vi "Labview_forward_pass.vi"() -> ()   [LabVIEW 2020]
uses:
  <vilib>/Analysis/NI_AALBase.lvlib
  <vilib>/Analysis/Matrix/NI_Matrix.lvlib
  <vilib>/Analysis/baseanly.llb/Real Dot Product.vi
  <vilib>/Analysis/Matrix/Numeric/Conversions/Array To Matrix - RA2.vi
  <vilib>/Analysis/baseanly.llb/Vector x A.vi
panel:
  out "i":i32
  out "xx":dbl[](array[numeric])
  out "element out":dbl
  out "XY Graph 2":cluster{i32[], dbl[]}(graph)
  out "y":dbl
  out "Array":i32[](array[numeric])
  out "XY Graph":T1(graph)
  out "X":dbl[](graph)
  out "All input data":waveform(dbl)(graph)
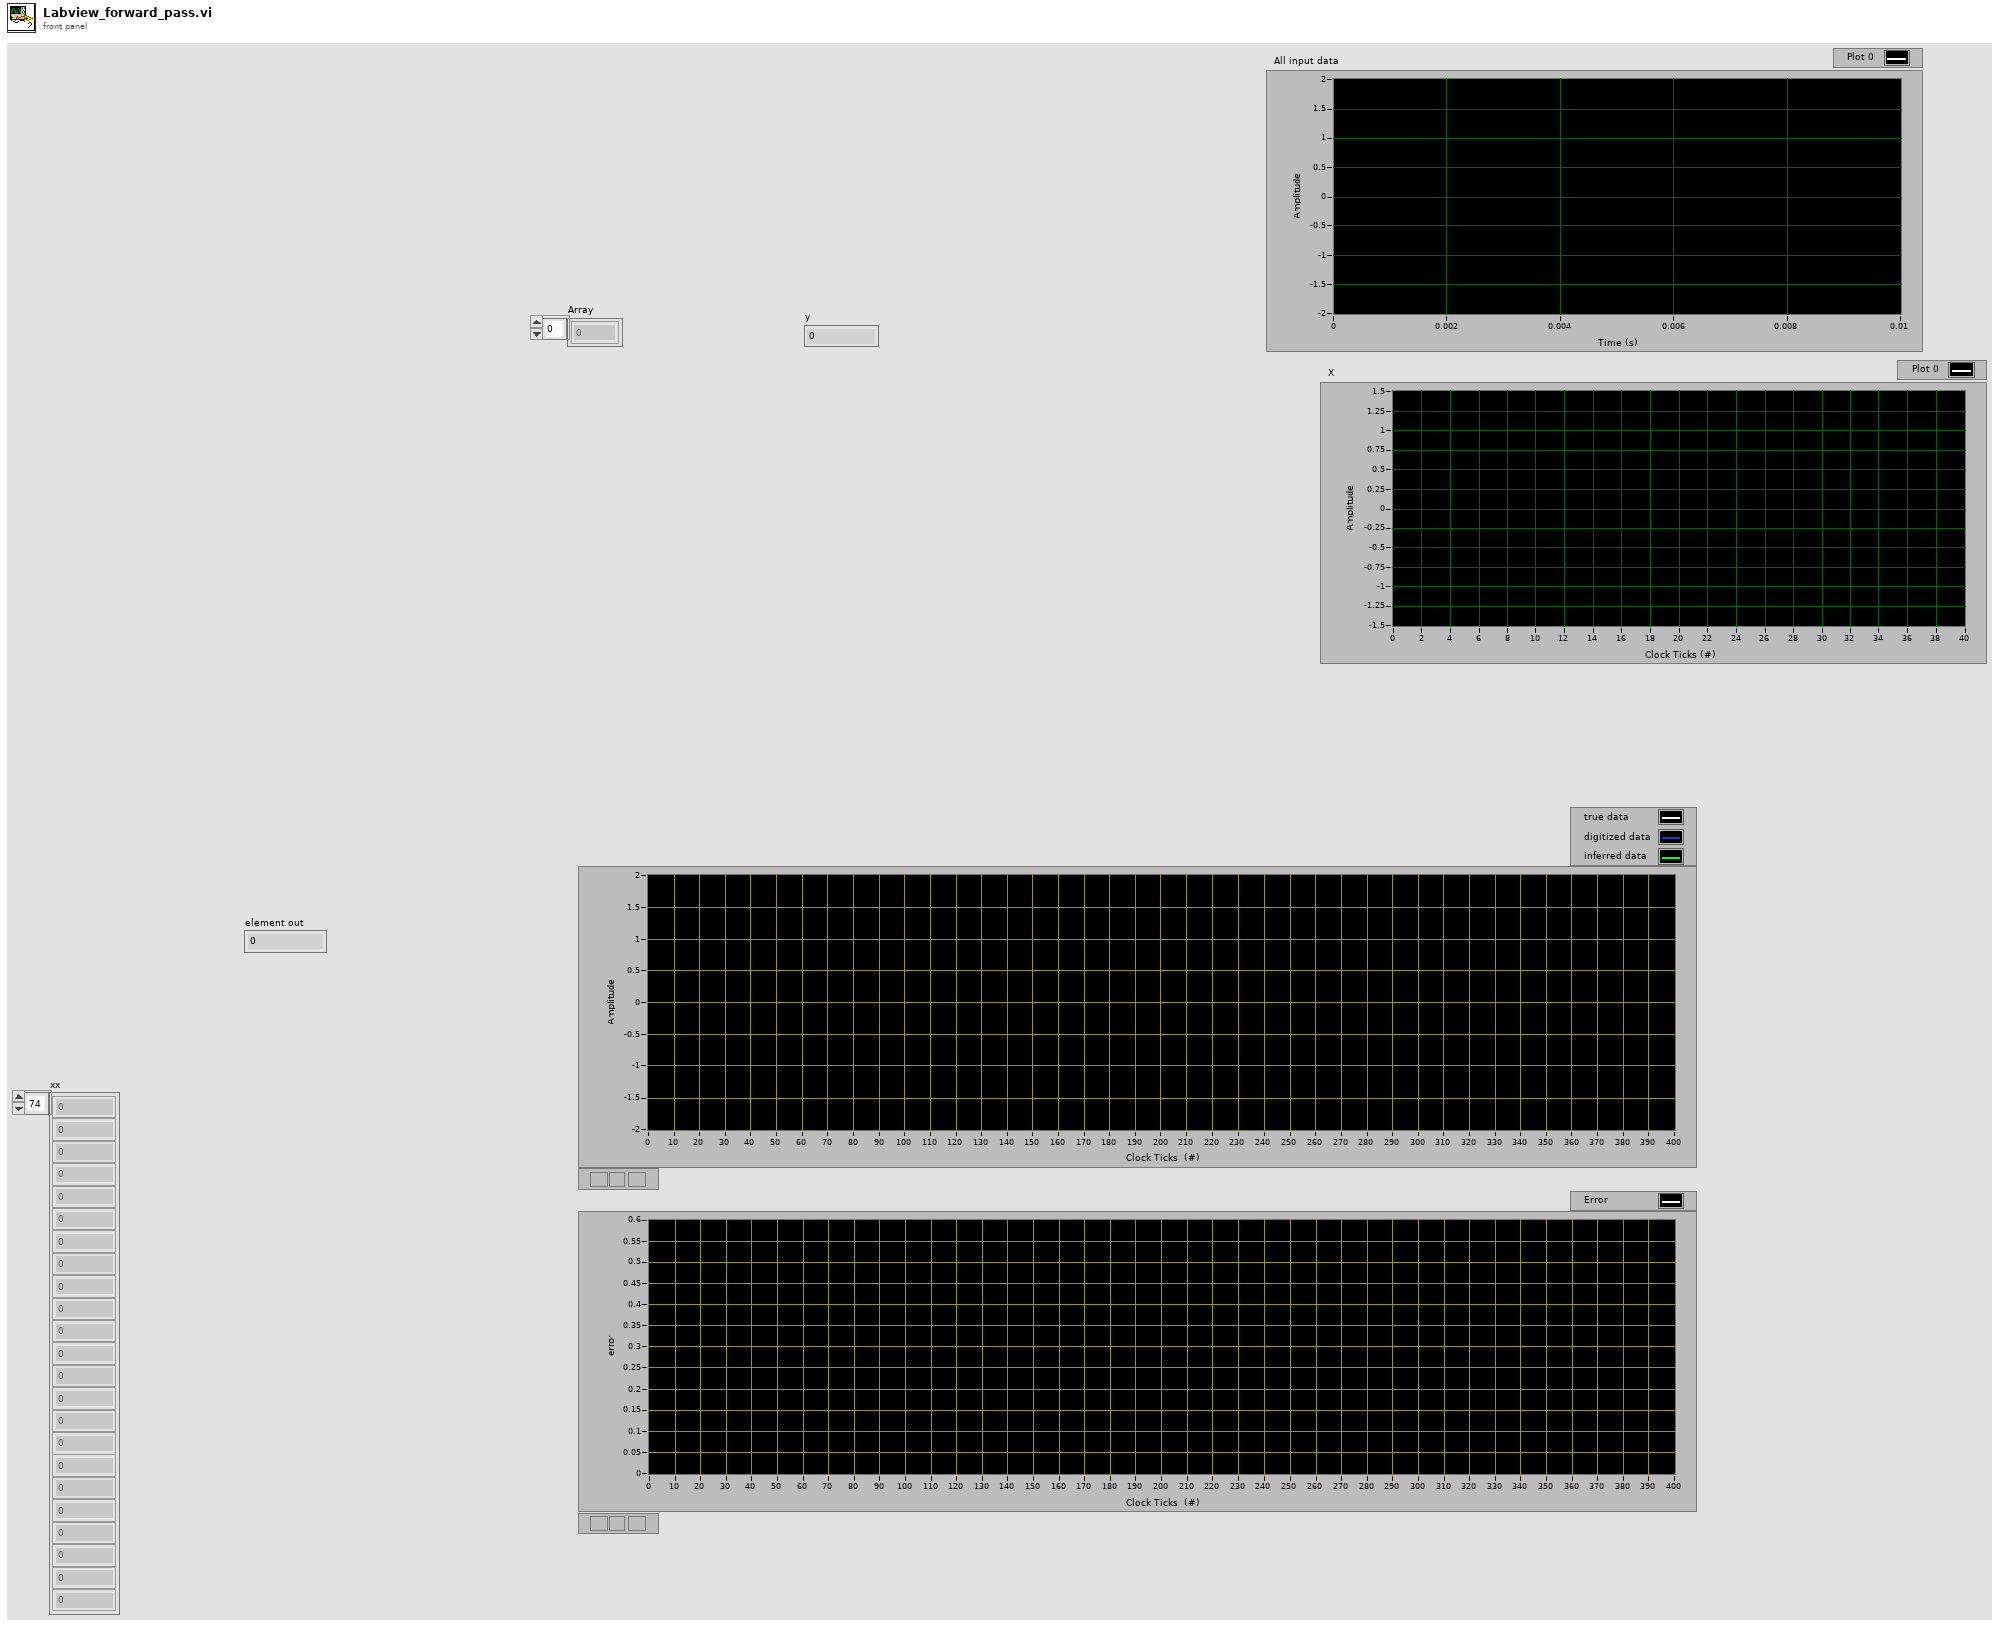
[diagram p1: front panel]
types:
  T1 = cluster{i32[], "array type (2D Dbl) out":dbl[]}[]
  T2 = typedef "NI_Matrix.lvlib/RealMatrix.ctl" = dbl[][]
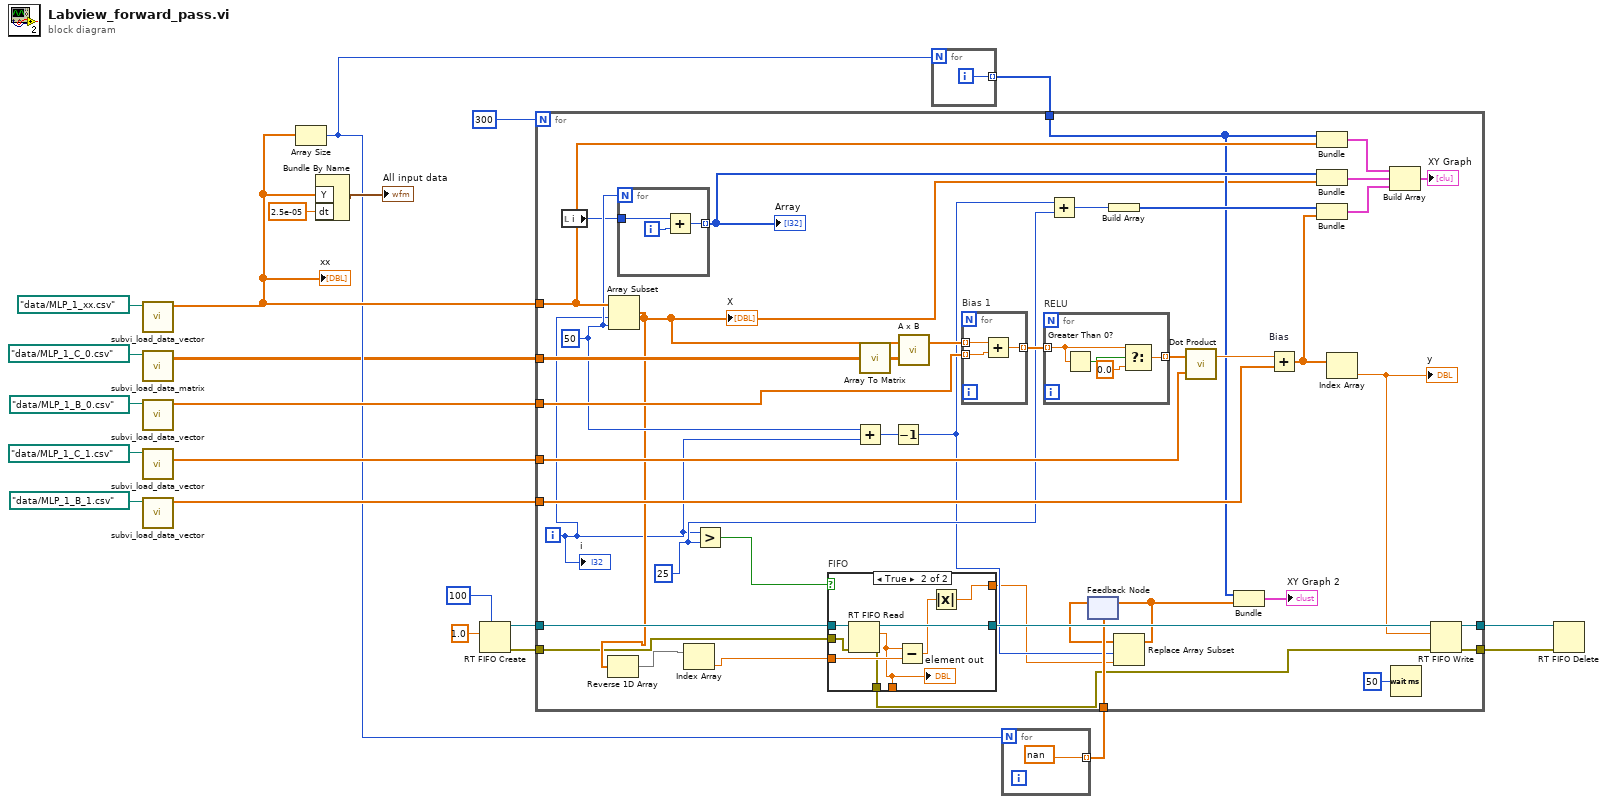
[diagram p0: block diagram]
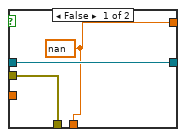
[diagram p2: hidden frame]
diagram:
  n1 = call "subvi_load_data_vector.vi"("default name"=path "data/MLP_1_xx.csv") -> ("array type (2D Dbl) out"=w8:dbl[])  [unwired: 10 in]
  "xx" <- w8
  n2 = call "subvi_load_data_matrix.vi"("default name"=path "data/MLP_1_C_0.csv") -> ("array"=w1:dbl[][])  [unwired: 10 in]
  n3 = call "subvi_load_data_vector.vi"("default name"=path "data/MLP_1_B_0.csv") -> ("array type (2D Dbl) out"=w15:dbl[])  [unwired: 10 in]
  n4 = call "subvi_load_data_vector.vi"("default name"=path "data/MLP_1_C_1.csv") -> ("array type (2D Dbl) out"=w16:dbl[])  [unwired: 10 in]
  n5 = call "subvi_load_data_vector.vi"("default name"=path "data/MLP_1_B_1.csv") -> ("array type (2D Dbl) out"=w14:dbl[])  [unwired: 10 in]
  n6 = Array Size(array=w8) -> (size(s)=w4:i32)
  n7 = Bundle By Name("Y"=w8, "dt"=2.5e-05) -> (→"All input data":waveform(dbl))  [unwired: 1 in]
  n8 = RT FIFO Create(1:1.0 ("dt"), 4:u32 100 ("size (10)")) -> (8:w5:refnum<k33>, 11:w3:errorcluster)  [unwired: 6 in, 1 out]
  n9 = for {
    N: w4 -> [_]
    tunnel: [w23] -> w11 mode=indexing
    i -> [w23]
  }
  n10 = for {
    N: w4 -> [_]
    tunnel: [nan] -> w9 mode=indexing
  }
  n11 = for {
    N: 300 -> [_]
    tunnel: w16 -> [w61]
    tunnel: w15 -> [w60]
    tunnel: w14 -> [w59]
    tunnel: w1 -> [w58]
    tunnel: w8 -> [w54]
    tunnel: w11 -> [w43]
    tunnel: w5 -> [w47]
    tunnel: [w45] -> w6
    tunnel: w9 -> [w41]
    tunnel: w3 -> [w28]
    tunnel: [w26] -> w2
    i -> [w25]
    w37 = 25 ("y")
    w38 = 50 ("length")
    n12 = local read "i"() -> (w29:i32)
    n13 = Array Subset(array=w54, index=w25, length=w38) -> (w34:dbl[])
    "X" <- w34
    n14 = Reverse 1D Array(array=w34) -> (reversed array=w33:dbl[])
    n15 = for {
      N: w38 -> [_]
      tunnel: w29 -> [w79]
      tunnel: [w78] -> w57 mode=indexing
      i -> [w80]
      n16 = Add(x=w79, y=w80) -> (x+y=w78:i32)
    }
    "Array" <- w57
    n17 = Index Array(array=w33) -> (element=w32:dbl)  [unwired: 1 in]
    n18 = Greater?(x=w25, y=w37) -> (0:w46:bool)
    n19 = case "FIFO" shown="True" w46 {
      tunnel: w47 -> [w69 w77]
      tunnel: [w69 w76] -> w44
      tunnel: [w68 w75] -> w30
      tunnel: w32 -> [_ w73]
      tunnel: [w68 w72] -> _
      tunnel: w28 -> [w67 w71]
      tunnel: [w67 w70] -> w27
      frame False {
        w68 = nan
      }
      frame True {
        n20 = RT FIFO Read(0:w77, 3:w71) -> (8:w76:refnum<k33>, 9:w72:dbl, 11:w70:errorcluster)  [unwired: 2 in, 2 out]
        "element out" <- w72
        n21 = Subtract(x=w72, y=w73) -> (x-y=w74:dbl)
        n22 = Absolute Value(x=w74) -> (abs(x)=w75:dbl)
      }
    }
    n23 = Add(x=w38, y=w25) -> (x+y=w36:i32)
    n24 = call-poly <vilib>:"Array To Matrix.vi"("Real 2D Array"=w58) -> ("Real Matrix"=w64:T2)
    n25 = Decrement(x=w36) -> (x-1=w35:i32)
    n26 = call-poly <vilib>:"A x B.vi"("Matrix A"=w64, "Vector V'"=w34) -> ("V' x A"=w66:dbl[])  [unwired: 1 out]
    n27 = for "Bias 1" {
      tunnel: w66 -> [w87] mode=indexing
      tunnel: [w86] -> w65 mode=indexing
      tunnel: w60 -> [w85] mode=indexing
      n28 = Add(x=w87, y=w85) -> (x+y=w86:dbl)
    }
    n29 = for "RELU" {
      tunnel: w65 -> [w84] mode=indexing
      tunnel: [w83] -> w63 mode=indexing
      n30 = Greater Than 0?(x=w84) -> (x > 0?=w81:bool)
      n31 = Select(t=w84, s=w81, f=0.0) -> (s? t:f=w83:dbl)
    }
    n32 = Add(x=w35, y=w37) -> (x+y=w52:i32)
    n33 = feedback #1(w41) -> (w39:dbl[])
    n34 = Build Array(w52) -> (w51:i32[])
    n35 = Replace Array Subset(array=w39, new element=w30, index=w35) -> (w40:dbl[])
    n36 = feedback-in #1(w40) -> ()
    n37 = call-poly <vilib>:"Dot Product.vi"("Y Vector"=w61, "X Vector"=w63) -> ("X * Y"=w62:dbl)  [unwired: 1 out]
    n38 = Bundle(w43, w40) -> (→"XY Graph 2":cluster{i32[], dbl[]})  [unwired: 1 in]
    n39 = Add "Bias"(x=w62, y=w59) -> (x+y=w53:dbl[])
    n40 = Bundle(w43, "array type (2D Dbl) out"=w54) -> (w48:cluster{i32[], "array type (2D Dbl) out":dbl[]})  [unwired: 1 in]
    n41 = Bundle(w57, w34) -> (w56:cluster{i32[], dbl[]})  [unwired: 1 in]
    n42 = Bundle(w51, w53) -> (w49:cluster{i32[], dbl[]})  [unwired: 1 in]
    n43 = Index Array(array=w53) -> (element=w31:dbl)  [unwired: 1 in]
    "y" <- w31
    n44 = Build Array(w48, w56, w49) -> (→"XY Graph":T1)
    n45 = Wait (ms)(milliseconds to wait=u32 50) -> ()  [unwired: 1 out]
    n46 = RT FIFO Write(0:w44, 1:w31, 3:w27) -> (8:w45:refnum<k33>, 11:w26:errorcluster)  [unwired: 2 in, 2 out]
    "i" <- w25
  }
  n47 = RT FIFO Delete(0:w6, 3:w2) -> ()  [unwired: 1 in, 1 out]
